vi "init.vi"(0 "Multi Analog Input Voltage Test in":refnum<class "Multi Analog Input Voltage Test.lvclass">, 1 "AO Voltage Data":T6 {"Bias" min=0.0 max=10.0 format="%.3f"; "NI Scaling" min=0.0 max=10.0 format="%.3f"; "Vref" min=0.0 max=10.0 format="%.3f"}, 2 "Multichannel Analog Input Test":T3 {"Tolerance" format="%.9f"; "Test Values"."Stop Value" format="%.6f"; "Test Values"."Start Value" format="%.6f"; "PGA Gain Coefficients" max=7}, 3 "Samples To Average":i32, 4 "ILC":refnum<class "ILC.lvclass">, 5 "error in (no error)":errorcluster, 6 "Delay Between Test Steps":u16, 7 "Log":refnum<class "ITestLog.lvclass">, 8 "CH24 DAQ Channel to Write":refnum<k21>, 9 "Scenario":T2, 10 "CH13 DAQ Channel to Write":refnum<k21>, 11 "Input Channels":T1) -> (14 "Multi Analog Input Voltage Test out":refnum<class "Multi Analog Input Voltage Test.lvclass">, 19 "error out":errorcluster)   [LabVIEW 2015, in "Multi Analog Input Voltage Test.lvclass"]
uses:
  Multi Analog Input Voltage Test.lvclass
  Typedefs/AI Voltage to NI Voltage.ctl
  Typedefs/Multichannel Analog Input Test.ctl
  <userlib>/Common/ILC/Configuration/ScanRate_Hz_MultichannelOptions.ctl
  Typedefs/Test Values.ctl
  Model/TestLog/ITestLog/ITestLog.lvclass
  <userlib>/Common/ILC/ILC/ILC.lvclass
  Typedefs/TestScenarioTypes.ctl
  <userlib>/Common/ILC/Configuration/InputChannels.ctl
  Multi Analog Input Voltage Test.lvclass/Multi Analog Input Voltage Test.ctl
  Typedefs/ILCBTTypedefs.lvlib
  <userlib>/Common/ILC/Configuration/ILCConfiguration.lvlib
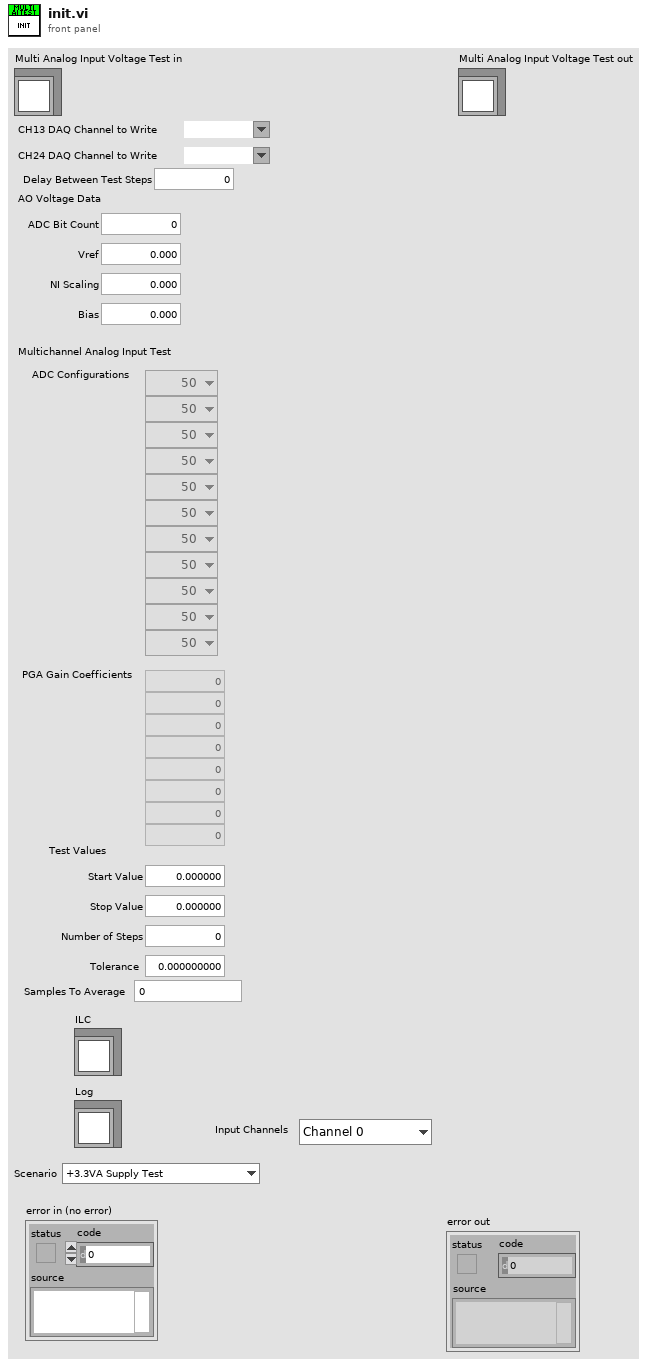
[diagram p1: front panel]
types:
  T1 = typedef "ILCCommon.lvlib/ILCConfiguration.lvlib/InputChannels.ctl" = enum16{"Channel 0", "3 Channels", "5 Channels"}
  T2 = typedef "ILCBTTypedefs.lvlib/TestScenarioTypes.ctl" = enum16{"+3.3VA Supply Test", "+3.3VD Supply Test", "+5VA Supply Test", "+5VD Supply Test", "Unique ID Test", "TEDS Status Test", "LIMSW1_TTL Low Test", "LIMSW1_TTL High Test", "LIMSW2_TTL Low Test", "LIMSW2_TTL High Test", "Tachometer Low Test", "Tachometer High Test", "SSR_TTL Low Test", "SSR_TTL High Test", "SM_GPI Low Test", "SM_GPI High Test", "CW Motion Without Limit Test", "CW Motion With Limit Test", "CW Motion With Both Limits Test", "CW Motion on CCW Limit Test", "CCW Motion Without Limit Test", "CCW Motion With Limit Test", "CCW Motion With Both Limits Test", "CCW Motion on CW Limit Test", "RS232-TXD Low Test", "RS232-TXD High Test", "RS232-RTS Low Test", "RS232-RTS High Test", "RS232-RXD Low Test", "RS232-RXD High Test", "RS232-CTS Low Test", "RS232-CTS High Test", "Out_SS Low Test", "Out_SS High Test", "Out_SDI Low Test", "Out_SDI High Test", "Out_SCLK Low Test", "Out_SCLK High Test", "Reset Low Test", "Reset High Test", "1 Channel ADC Test", "3 Channel ADC Test", "5 Channel ADC Test", "Vref Test", "ROT Test", "DAC1 Test", "DAC2 Test", "DAC3 Test", "DAC4 Test", "BIAS Test", "EXC1 Test", "EXC2 Test", "EXC3 Test", "EXC4 Test"}
  T3 = typedef "ILCBTTypedefs.lvlib/Multichannel Analog Input Test.ctl" = cluster{"ADC Configurations":T4[], "PGA Gain Coefficients":u16[], "Test Values":T5, "Tolerance":dbl}
  T4 = typedef "ILCCommon.lvlib/ILCConfiguration.lvlib/ScanRate_Hz_MultichannelOptions.ctl" = enum16{"50", "60", "100", "120", "200", "240", "300", "400", "480", "600", "1200", "2400", "4800"}
  T5 = typedef "ILCBTTypedefs.lvlib/Test Values.ctl" = cluster{"Start Value":dbl, "Stop Value":dbl, "Number of Steps":u16}
  T6 = typedef "ILCBTTypedefs.lvlib/AI Voltage to NI Voltage.ctl" = cluster{"ADC Bit Count":u16, "Vref":dbl, "NI Scaling":dbl, "Bias":dbl}
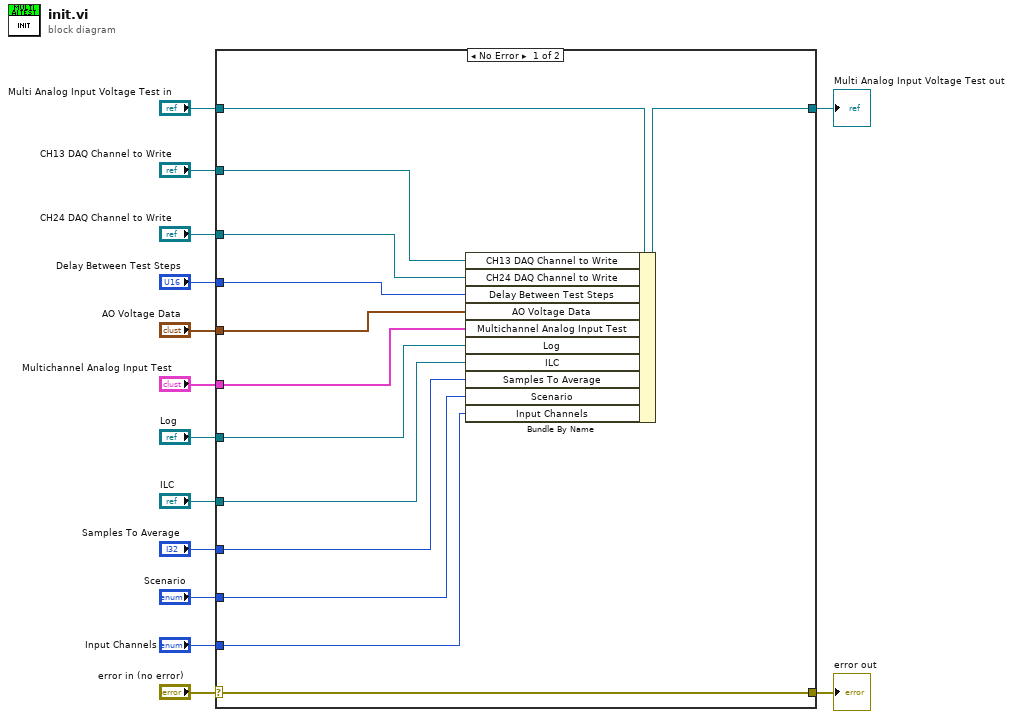
[diagram p0: block diagram]
diagram:
  n1 = case shown="No Error" "error in (no error)" {
    selector: "error in (no error)" -> [w27 w29]
    tunnel: [w27 w29] -> w13
    tunnel: [w25 w28] -> w11
    tunnel: "Multi Analog Input Voltage Test in" -> [w26 w28]
    tunnel: "CH13 DAQ Channel to Write" -> [w24 _]
    tunnel: "CH24 DAQ Channel to Write" -> [w23 _]
    tunnel: "Delay Between Test Steps" -> [w22 _]
    tunnel: "AO Voltage Data" -> [w21 _]
    tunnel: "Multichannel Analog Input Test" -> [w20 _]
    tunnel: "ILC" -> [w19 _]
    tunnel: "Log" -> [w18 _]
    tunnel: "Samples To Average" -> [w17 _]
    tunnel: "Scenario" -> [w16 _]
    tunnel: "Input Channels" -> [w15 _]
    frame No Error {
      n2 = Bundle By Name(cluster=w26, "CH13 DAQ Channel to Write"=w24, "CH24 DAQ Channel to Write"=w23, "Delay Between Test Steps"=w22, "AO Voltage Data"=w21, "Multichannel Analog Input Test"=w20, "Log"=w18, "ILC"=w19, "Samples To Average"=w17, "Scenario"=w16, "Input Channels"=w15) -> (w25:refnum<class "Multi Analog Input Voltage Test.lvclass">)
    }
    frame Error {
    }
  }
  "error out" <- w13
  "Multi Analog Input Voltage Test out" <- w11
